vi "%s (Request).vi"(8 "error in (no error)":errorcluster, 11 "API in":refnum<class "Interface.lvclass">) -> (0 "error out":errorcluster, 3 "API out":refnum<class "Interface.lvclass">)   [LabVIEW 2018, in "Scripting.lvlib" / "Actor.lvlib" / "Interface.lvclass"]
uses:
  Interface.lvclass
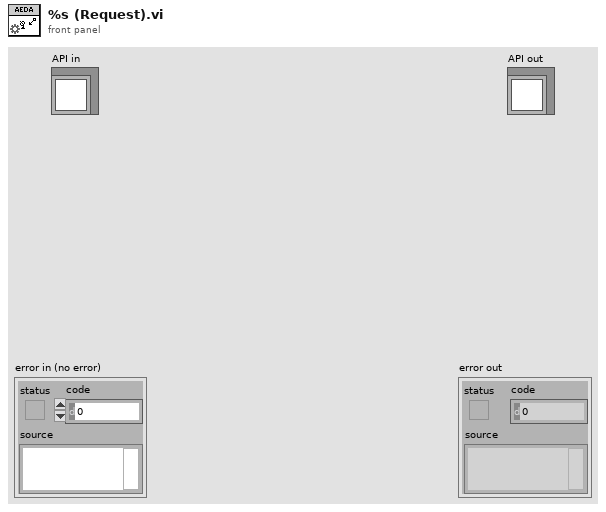
[diagram p1: front panel]
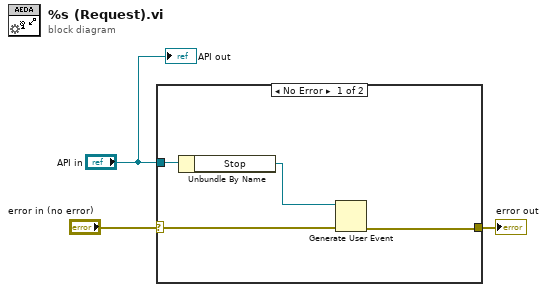
[diagram p0: block diagram]
diagram:
  n1 = case shown="No Error" "error in (no error)" {
    selector: "error in (no error)" -> [w7 w8]
    tunnel: [w6 w8] -> w2
    tunnel: "API in" -> [w4 _]
    frame No Error {
      n2 = Unbundle By Name(w4) -> ("Stop"=w5:refnum<user-event>)
      n3 = Generate User Event(user event=w5, error in=w7) -> (error out=w6:errorcluster)  [unwired: 2 in, 1 out]
    }
    frame Error {
    }
  }
  "error out" <- w2
  "API out" <- "API in"
